vi "ConfigureSimulatedHardware.vi"(8 "error in (no error)":errorcluster, 11 "Scan Engine Config":T1) -> (0 "error out":errorcluster, 3 "Scan Engine Config Out":T1)   [LabVIEW 2017, in "ScanEngine.lvlib"]
uses:
  <vilib>/addons/InsightCM/Devices/Shared/Common/ScanEngine/ScanEngine.lvlib
  <vilib>/addons/InsightCM/Devices/Shared/Common/ScanEngine/controls/Configuration.ctl
  <vilib>/addons/InsightCM/Devices/Shared/Common/ScanEngine/controls/Group.ctl
  <vilib>/addons/InsightCM/Devices/Shared/Common/ScanEngine/controls/Channel.ctl
  <vilib>/Utility/Data Type/Type Definitions/Data Type.ctl
  <vilib>/addons/InsightCM/MessageBus/Base/controls/KeyValuePair.ctl
  <vilib>/addons/InsightCM/Devices/Shared/Common/ScanEngine/controls/SimulatedData.ctl
  <vilib>/addons/InsightCM/Devices/Shared/Common/ScanEngine/subVIs/SimulatedConfigRefGlobal.vi
  <vilib>/Utility/Data Type/NI_Data Type.lvlib
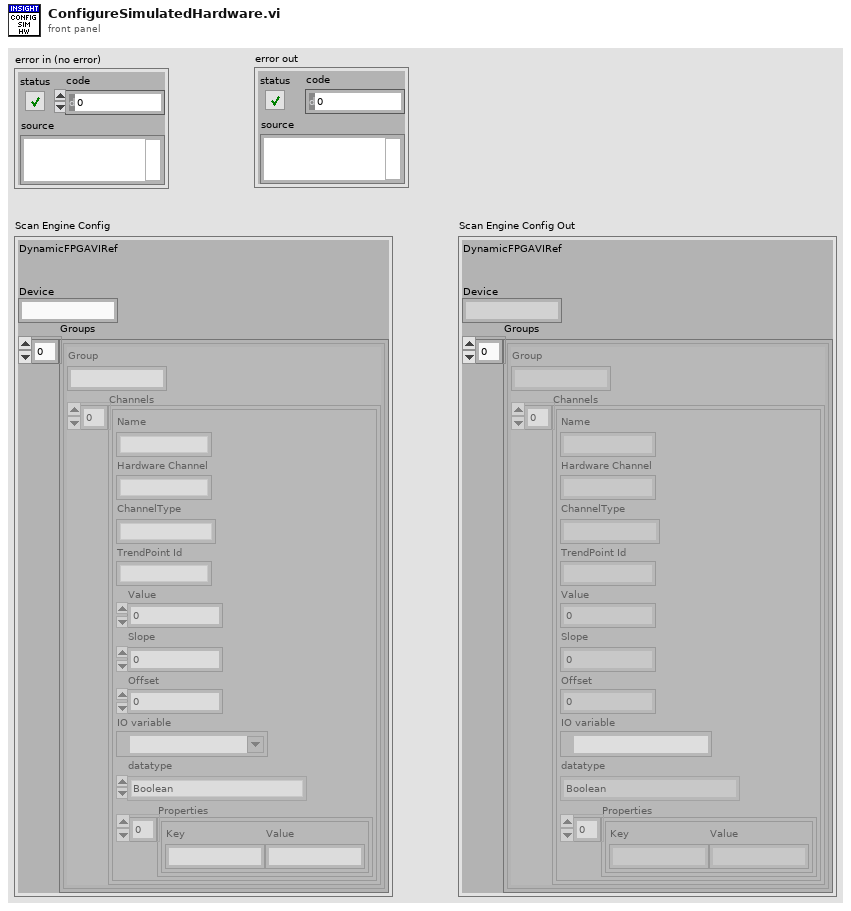
[diagram p1: front panel]
types:
  T1 = typedef "ScanEngine.lvlib/Configuration.ctl" = cluster{"DynamicFPGAVIRef":refnum<k20>, "Device":string, "Groups":T2[]}
  T2 = typedef "ScanEngine.lvlib/Group.ctl" = cluster{"Group":string, "Channels":T3[]}
  T3 = typedef "ScanEngine.lvlib/Channel.ctl" = cluster{"Name":string, "Hardware Channel":string, "ChannelType":string, "TrendPoint Id":string, "Value":sgl, "Slope":dbl, "Offset":dbl, "IO variable":refnum<k21>, "datatype":T4, "Properties":T5[]}
  T4 = typedef "NI_Data Type.lvlib/Data Type.ctl" = enum8{"Invalid Type", "Void", "I8", "I16", "I32", "I64", "U8", "U16", "U32", "U64", "Single Float", "Double Float", "Extended Float", "Single Complex", "Double Complex", "Extended Complex", "Enum U8", "Enum U16", "Enum U32", "Enum U64", "Single Float With Unit", "Double Float With Unit", "Extended Float With Unit", "Single Complex with Unit", "Double Complex with Unit", "Extended Complex with Unit", "Boolean", "String", "Path", "Picture", "Tag", "Array", "Cluster", "Variant", "LV Variant", "Waveform", "Timestamp", "Digital Waveform", "Digital Data", "ExpressData", "Refnum", "External Data", "VI", "Poly VI", "LabVIEW Class Instance", "Fixed Point"}
  T5 = typedef "KeyValuePair.ctl" = cluster{"Key":string, "Value":string}
  T6 = typedef "ScanEngine.lvlib/SimConfigRefs.ctl" = cluster{"Scan Engine Config":refnum<vi>}
  T7 = typedef "ScanEngine.lvlib/SimulatedData.ctl" = cluster{"Channel":string, "Value":dbl, "Random":bool, "Delta":dbl}
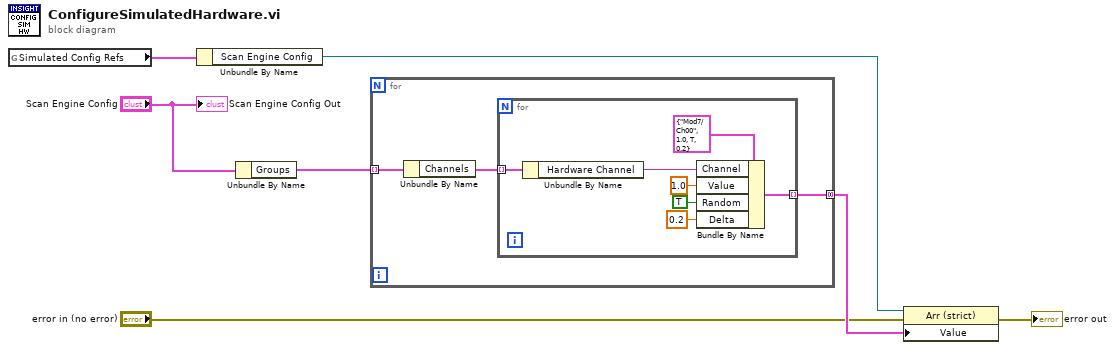
[diagram p0: block diagram]
diagram:
  n1 = global read "SimulatedConfigRefGlobal.vi" "Simulated Config Refs"() -> (w1:T6)
  n2 = Unbundle By Name(w1) -> ("Scan Engine Config"=w6:refnum<vi>)
  n3 = Unbundle By Name("Scan Engine Config") -> ("Groups"=w2:T2[])
  n4 = for {
    tunnel: [w10] -> w7 mode=concatenating
    tunnel: w2 -> [w9] mode=indexing
    n5 = Unbundle By Name(w9) -> ("Channels"=w8:T3[])
    n6 = for {
      tunnel: w8 -> [w17] mode=indexing
      tunnel: [w12] -> w10 mode=indexing
      n7 = Unbundle By Name(w17) -> ("Hardware Channel"=w16:string)
      n8 = Bundle By Name(cluster=T7 {"Channel"="Mod7/Ch00", "Value"=1.0, "Random"=TRUE, "Delta"=0.2} ("Cluster"), "Channel"=w16, "Value"=1.0, "Random"=TRUE, "Delta"=0.2) -> (w12:T7)
    }
  }
  n9 = property class="Arr (strict)"(reference=w6, error in="error in (no error)", "Value"=w7) -> (error out=→"error out":errorcluster)  [unwired: 1 out]
  "Scan Engine Config Out" <- "Scan Engine Config"
